vi "GetFeedforward.vi"(11 "scope in":T1) -> (1 "values Q":dbl[](array[numeric]), 2 "values I":dbl[](array[numeric]), 3 "scope out":T1)   [LabVIEW 2013]
uses:
  controls/scope_params_5782.ctl
  Utilities/Ticker/Ticker.lvclass
  Communication/Driver/RemoteConnection/RemoteConnection.lvclass
  Scope/controls/ScopeMode.ctl
  Config/FPGAref_5782.ctl
  FPGA/DataMode.ctl
  controls/5782_trigger_type.ctl
  controls/Feedforward.ctl
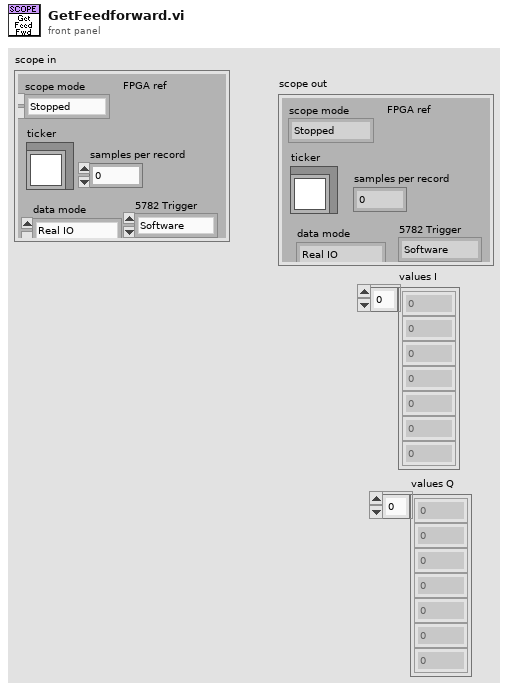
[diagram p1: front panel]
types:
  T1 = typedef "scope_params_5782.ctl" = cluster{"scope mode":T2, "ticker":refnum<class "Ticker.lvclass">, "samples per record":i32, "FPGA ref":T3, "data mode":T4, "5782 Trigger":T5, "Chart length":i32, "RemoteConnection":refnum<class "RemoteConnection.lvclass">, "last phase":dbl[], "Feedforward":T6}
  T2 = typedef "ScopeMode.ctl" = enum16{"Stopped", "Single", "Running", "Continuous"}
  T3 = typedef "FPGAref_5782.ctl" = refnum<k20>
  T4 = typedef "DataMode.ctl" = enum16{"Real IO", "Simulated"}
  T5 = typedef "5782_trigger_type.ctl" = enum16{"Software", "Trigger input"}
  T6 = typedef "Feedforward.ctl" = cluster{"Beam I":dbl[], "Beam Q":dbl[], "Feedforward I":dbl[], "Feedforward Q":dbl[], "Setpoint I":dbl[], "Setpoint Q":dbl[]}
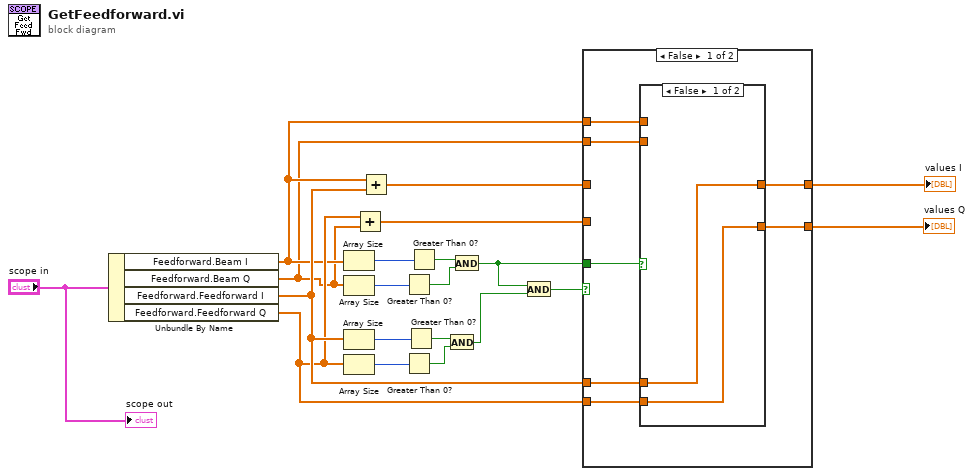
[diagram p0: block diagram]
diagram:
  n1 = Unbundle By Name("scope in") -> ("Feedforward.Beam I"=w3:dbl[], "Feedforward.Beam Q"=w2:dbl[], "Feedforward.Feedforward I"=w5:dbl[], "Feedforward.Feedforward Q"=w4:dbl[])
  n2 = Array Size(array=w3) -> (size(s)=w20:i32)
  n3 = Array Size(array=w2) -> (size(s)=w19:i32)
  n4 = Array Size(array=w5) -> (size(s)=w17:i32)
  n5 = Array Size(array=w4) -> (size(s)=w18:i32)
  n6 = Add(x=w4, y=w2) -> (x+y=w9:dbl[])
  n7 = Add(x=w3, y=w5) -> (x+y=w10:dbl[])
  n8 = Greater Than 0?(x=w19) -> (x > 0?=w15:bool)
  n9 = Greater Than 0?(x=w18) -> (x > 0?=w13:bool)
  n10 = Greater Than 0?(x=w17) -> (x > 0?=w14:bool)
  n11 = Greater Than 0?(x=w20) -> (x > 0?=w16:bool)
  n12 = And(x=w14, y=w13) -> (x .and. y?=w12:bool)
  n13 = And(x=w16, y=w15) -> (x .and. y?=w6:bool)
  n14 = And(x=w6, y=w12) -> (x .and. y?=w11:bool)
  n15 = case shown="False" w11 {
    tunnel: w10 -> [_ w32]
    tunnel: w9 -> [_ w33]
    tunnel: [w21 w33] -> w7
    tunnel: [w22 w32] -> w8
    tunnel: w6 -> [w27 _]
    tunnel: w5 -> [w26 _]
    tunnel: w4 -> [w25 _]
    tunnel: w3 -> [w24 _]
    tunnel: w2 -> [w23 _]
    frame False {
      n16 = case shown="False" w27 {
        tunnel: w26 -> [w29 _]
        tunnel: w25 -> [w28 _]
        tunnel: w24 -> [_ w31]
        tunnel: w23 -> [_ w30]
        tunnel: [w29 w31] -> w22
        tunnel: [w28 w30] -> w21
        frame False {
        }
        frame True {
        }
      }
    }
    frame True {
    }
  }
  "values I" <- w8
  "values Q" <- w7
  "scope out" <- "scope in"
